vi "Parser.vi"(1 "string":string) -> (0 "Out Strings":string[](array[string]))   [LabVIEW 2014]
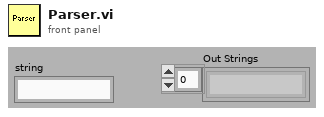
[diagram p1: front panel]
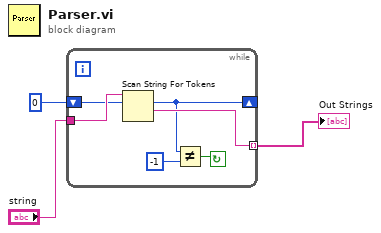
[diagram p0: block diagram]
diagram:
  n1 = while {
    tunnel: "string" -> [w9]
    shift-right: [w5] -> _
    shift-left: 0 ("offset past token") -> [w8]
    tunnel: [w7] -> w2 mode=indexing
    stop <- w6 continue-if-true
    n2 = Scan String For Tokens(8:w8, 9:w9) -> (1:w7:string, 2:w5:i32)  [unwired: 4 in, 2 out]
    n3 = Not Equal?(x=w5, y=-1) -> (x != y?=w6:bool)
  }
  "Out Strings" <- w2
